vi "NET SetInputShape.vi"(8 "error in (no error)":errorcluster, 9 "Shape":i32[](array[numeric]), 10 "InputName":string, 11 "NET in":refnum<class "NET.lvclass">) -> (0 "error out":errorcluster, 3 "NET out":refnum<class "NET.lvclass">)   [LabVIEW 2020, in "OpenLvVision_OpenCv.lvlib" / "NET.lvclass"]
doc: "Specify shape of network input."
uses:
  NET.lvclass
  C:/Users/lukas/Downloads/OpenLvVision_OpenCv/SourceCode/LabView/OpenLvVision_OpenCv/_LvHelpers/EdvrObject/EdvrObject.lvclass
  _LvHelpers/EdvrObject/EdvrObject.lvclass/EdvrObject.ctl
  OpenLvVision_OpenCv.lvlib
  _LvHelpers/EdvrObject/EdvrObject.lvclass
  Dlls/OlvOpenCvWrapper.dll
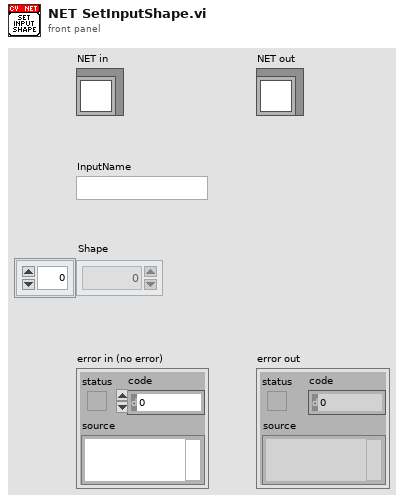
[diagram p1: front panel]
types:
  T1 = typedef "OpenLvVision_OpenCv.lvlib/EdvrObject.lvclass/Edvr.ctl" = refnum<data-value>
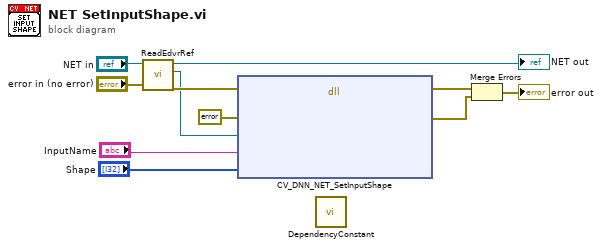
[diagram p0: block diagram]
diagram:
  n1 = call "ReadEdvrRef.vi"("error in (no error)"="error in (no error)", "EdvrObject in"="NET in") -> ("error out"=w7:errorcluster, "Edvr"=w6:T1, "EdvrObject out"=→"NET out":refnum<class "NET.lvclass">)  [unwired: 7 in]
  n2 = dll-call lib="C:/Users/lukas/Downloads/OpenLvVision_OpenCv/SourceCode/LabView/OpenLvVision_OpenCv/Dlls/OlvOpenCvWrapper.dll" fn="CV_DNN_NET_SetInputShape"(error in=w7, "Error"=errorcluster {"status"=FALSE, "code"=0, "source"=""} ("error out"), "edvrRef"=w6, "inputName"="InputName", "shape"="Shape") -> (error out=w10:errorcluster, "Error"=w3:errorcluster)  [unwired: 6 in, 1 out]
  n3 = call "DependencyConstant.vi"() -> ()  [unwired: 12 in]
  n4 = Merge Errors(w10, w3) -> (→"error out":errorcluster)
